vi "Set Stream Speed and Acceleration (Polymorphic).vi"   [LabVIEW 2013, in "Zaber A Series.lvlib"]
doc: "Change the maximum speed and acceleration parameters of an open stream. This command does not take effect until any other commands already in the stream have been completed.\n\nSpeed and accleration inputs are in device units. Use the Convert Velocity/Acceleration Units to Device Units VIs to convert from standard units of measure. A value of 0 for Maximum Speed, Tangential Acceleration, or Centripetal Acceleration will leave that property unchanged.\n\nThis VI does not check in advance for error conditions such as streams not being supported.\n\nThis VI requires that the Initialize VI has been called with the same serial port."
uses:
  Zaber A Series.lvlib
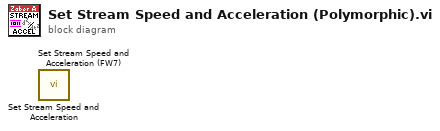
[diagram p0: block diagram]
diagram:
  n1 = call "Set Stream Speed and Acceleration.vi"() -> ()  [unwired: 10 in, 2 out]
  n2 = call "Set Stream Speed and Acceleration (FW7).vi"() -> ()  [unwired: 10 in, 2 out]
